vi "Odor_Control_b.vi"() -> ()   [LabVIEW 2014]
uses:
  <vilib>/Utility/file.llb/Read From Spreadsheet File (DBL).vi
  Image Aquisition - Labview/Image Recorder/experiment state global.vi
panel:
  in  "Sync Mode":bool
  out "Security Valve \nfor Mixtures":bool
  in  "threshold \nfor mixture":dbl
  in  "File with signal for odor 2":path=path "\\\\LABNAS40\\Luis/2016/Chemotaxis/Test/20160308/sine.txt"
  in  "File with signal for odor 1":path=path "\\\\LABNAS40\\Luis/2016/Chemotaxis/w1118_Acetal_1in250_50mfc/20160614/sine.txt"
  in  "ODOR 2":bool
  in  "ODOR 1":bool=TRUE
  in  "ODOR 2 FLOW %":dbl(slide) scale=0.0..100.0
  in  "ODOR 1 FLOW %":dbl(slide) scale=0.0..100.0
  in  "ODOR 2":bool
  in  "ODOR 1":bool=TRUE
  in  "TOLERANCE \nFOR CLOSING \nVALVE MANIFOLD":dbl=1.0
  in  "Serial Port":refnum<visa-resource-name>="COM3"
  in  "MODE SELECTOR":string(combo)="MANUAL"
  out "Path":path=path "B:/Luis/2016/0613/1047"
  in  "8":bool
  in  "7":bool
  in  "6":bool
  in  "5":bool
  in  "4":bool
  in  "3":bool
  in  "2":bool
  in  "1":bool
  in  "Start Recording":bool
  in  "extra label:":string="t101"
  in  "Save To:":path=path "B:/Luis"
  in  "CLEAR stored data":bool
  in  "Select signal to plot":T1(ring)=enum."odor 1 flow rate"
  out "XY Graph":T2(graph)
  in  "Air Flow Rate \n(L/min)":dbl
  in  "odor 2 between experiments":dbl
  in  "odor 2 signal parameters":T3={"temporal ramp type"=enum."Sine", "period(s)"=20.0, "high limit"=0.0, "low limit"=0.0, "duty cycle (sq wave)"=50.0} {"low limit" format="%#_6p"}
  in  "odor 1 between experiments":dbl
  in  "Sync Signal To \nImage Aquisition":bool
  in  "ENABLE MFCs":bool=TRUE
  in  "Restart Signal":bool
  in  "odor 1 signal parameters":T3={"temporal ramp type"=enum."Sine", "period(s)"=20.0, "high limit"=100.0, "low limit"=10.0, "duty cycle (sq wave)"=50.0} {"low limit" format="%#_6p"}
  in  "update period (ms)":u32=100
  in  "?":bool
  # "NOTE: Always start with Start Recording OFF, don't turn OFF while running"
  # "Manual Stop"
  # "VALVE CONTROL"
  # "MANUAL"
  # "FROM FILE"
  # "PREDEFINED WAVEFORM"
  # "PARAMETERS FOR BACKWASH PREVENTION"
  # "Only use when using odor \nmixture configuration, otherwise \nset to 0"
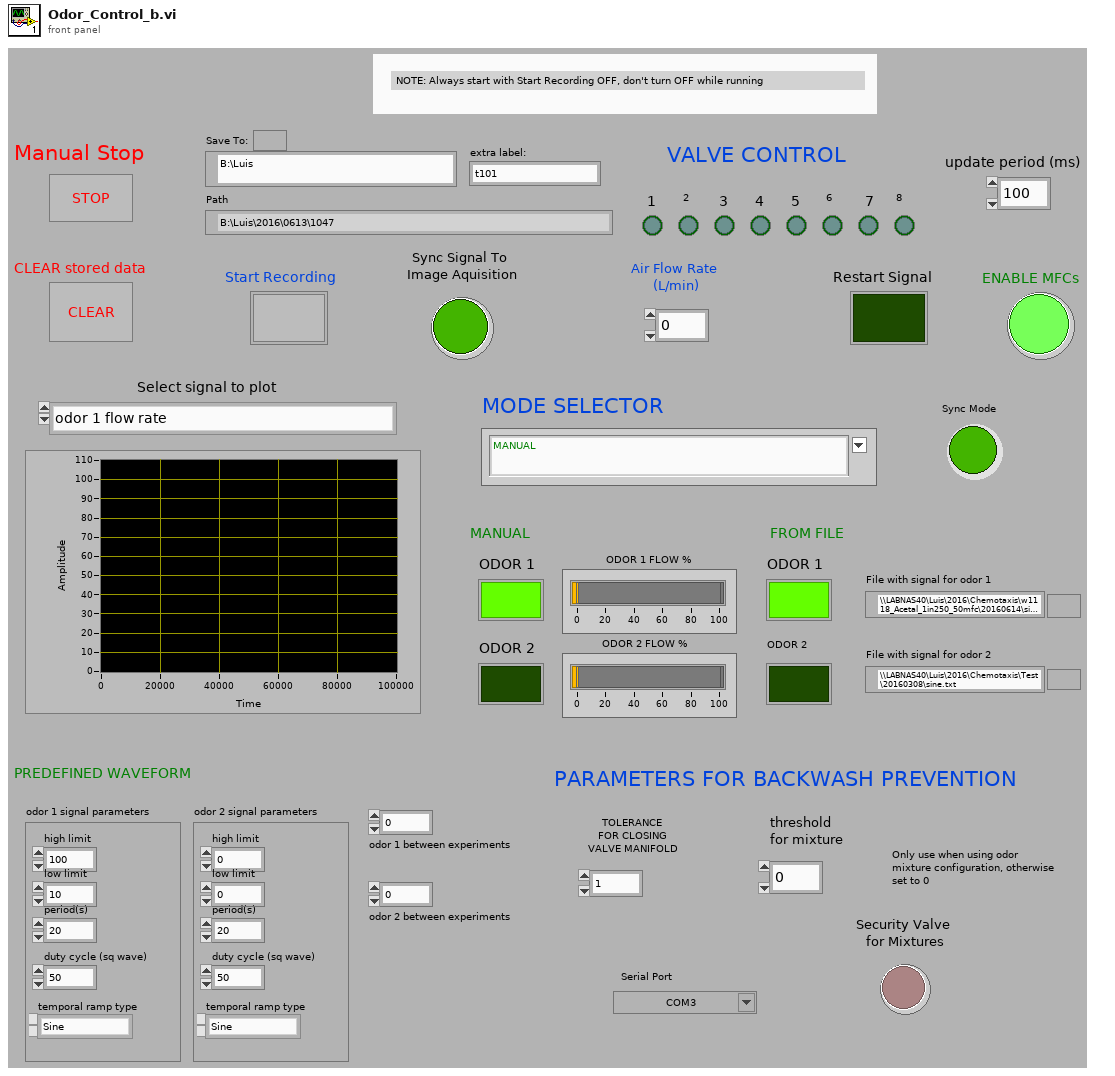
[diagram p1: front panel]
types:
  T1 = enum16{"air setpoint", "air flow rate", "odor 1 set point", "odor 1 flow rate", "odor 2 setpoint", "odor 2 flow rate", "pid reading", "led current", "led voltage", "led setpoint", "led temperature"}
  T2 = cluster{"Value Array":dbl[], "Value Array":dbl[]}
  T3 = cluster{"temporal ramp type":enum16{"Sine", "Triangle", "Sawtooth", "Square", "Exponential"}, "period(s)":dbl, "high limit":dbl, "low limit":dbl, "duty cycle (sq wave)":dbl}
  T4 = cluster{"analog output channels":cluster{"air ao":refnum<k21>, "odor 1 ao":refnum<k21>, "odor 2 ao":refnum<k21>}, "analog input channels":cluster{"air ai":refnum<k21>, "odor 1 ai":refnum<k21>, "odor 2 ai":refnum<k21>, "pid sensor 1 ai":refnum<k21>, "pid sensor 2 ai":refnum<k21>}, "digital control lines":cluster{"air close":refnum<k21>, "air purge":refnum<k21>, "odor 1 close":refnum<k21>, "odor 1 purge":refnum<k21>, "odor 2 close":refnum<k21>, "odor 2 purge":refnum<k21>}}
  T5 = enum16{"T - set Time per step", "N - set Number of valves", "F - turn gradient on Forward", "R - turn gradient on Reverse", "M - turn valves on 50% of time (mix)", "O - all valves Open (active)", "C - all valves Closed (inactive)", "V - set Valve state", "S - query valve State", "Q - Quiet (only error msgs)", "L - Loud (acknowledge all)", "H - useless Help message"}
  T6 = enum16{"Reset Table", "Get Values", "Add Value", "Get Table", "Get Spreadsheet", "set stack writer"}
  T7 = cluster{"experiment started":bool, "experiment ended":bool, "experiment start time":u32}
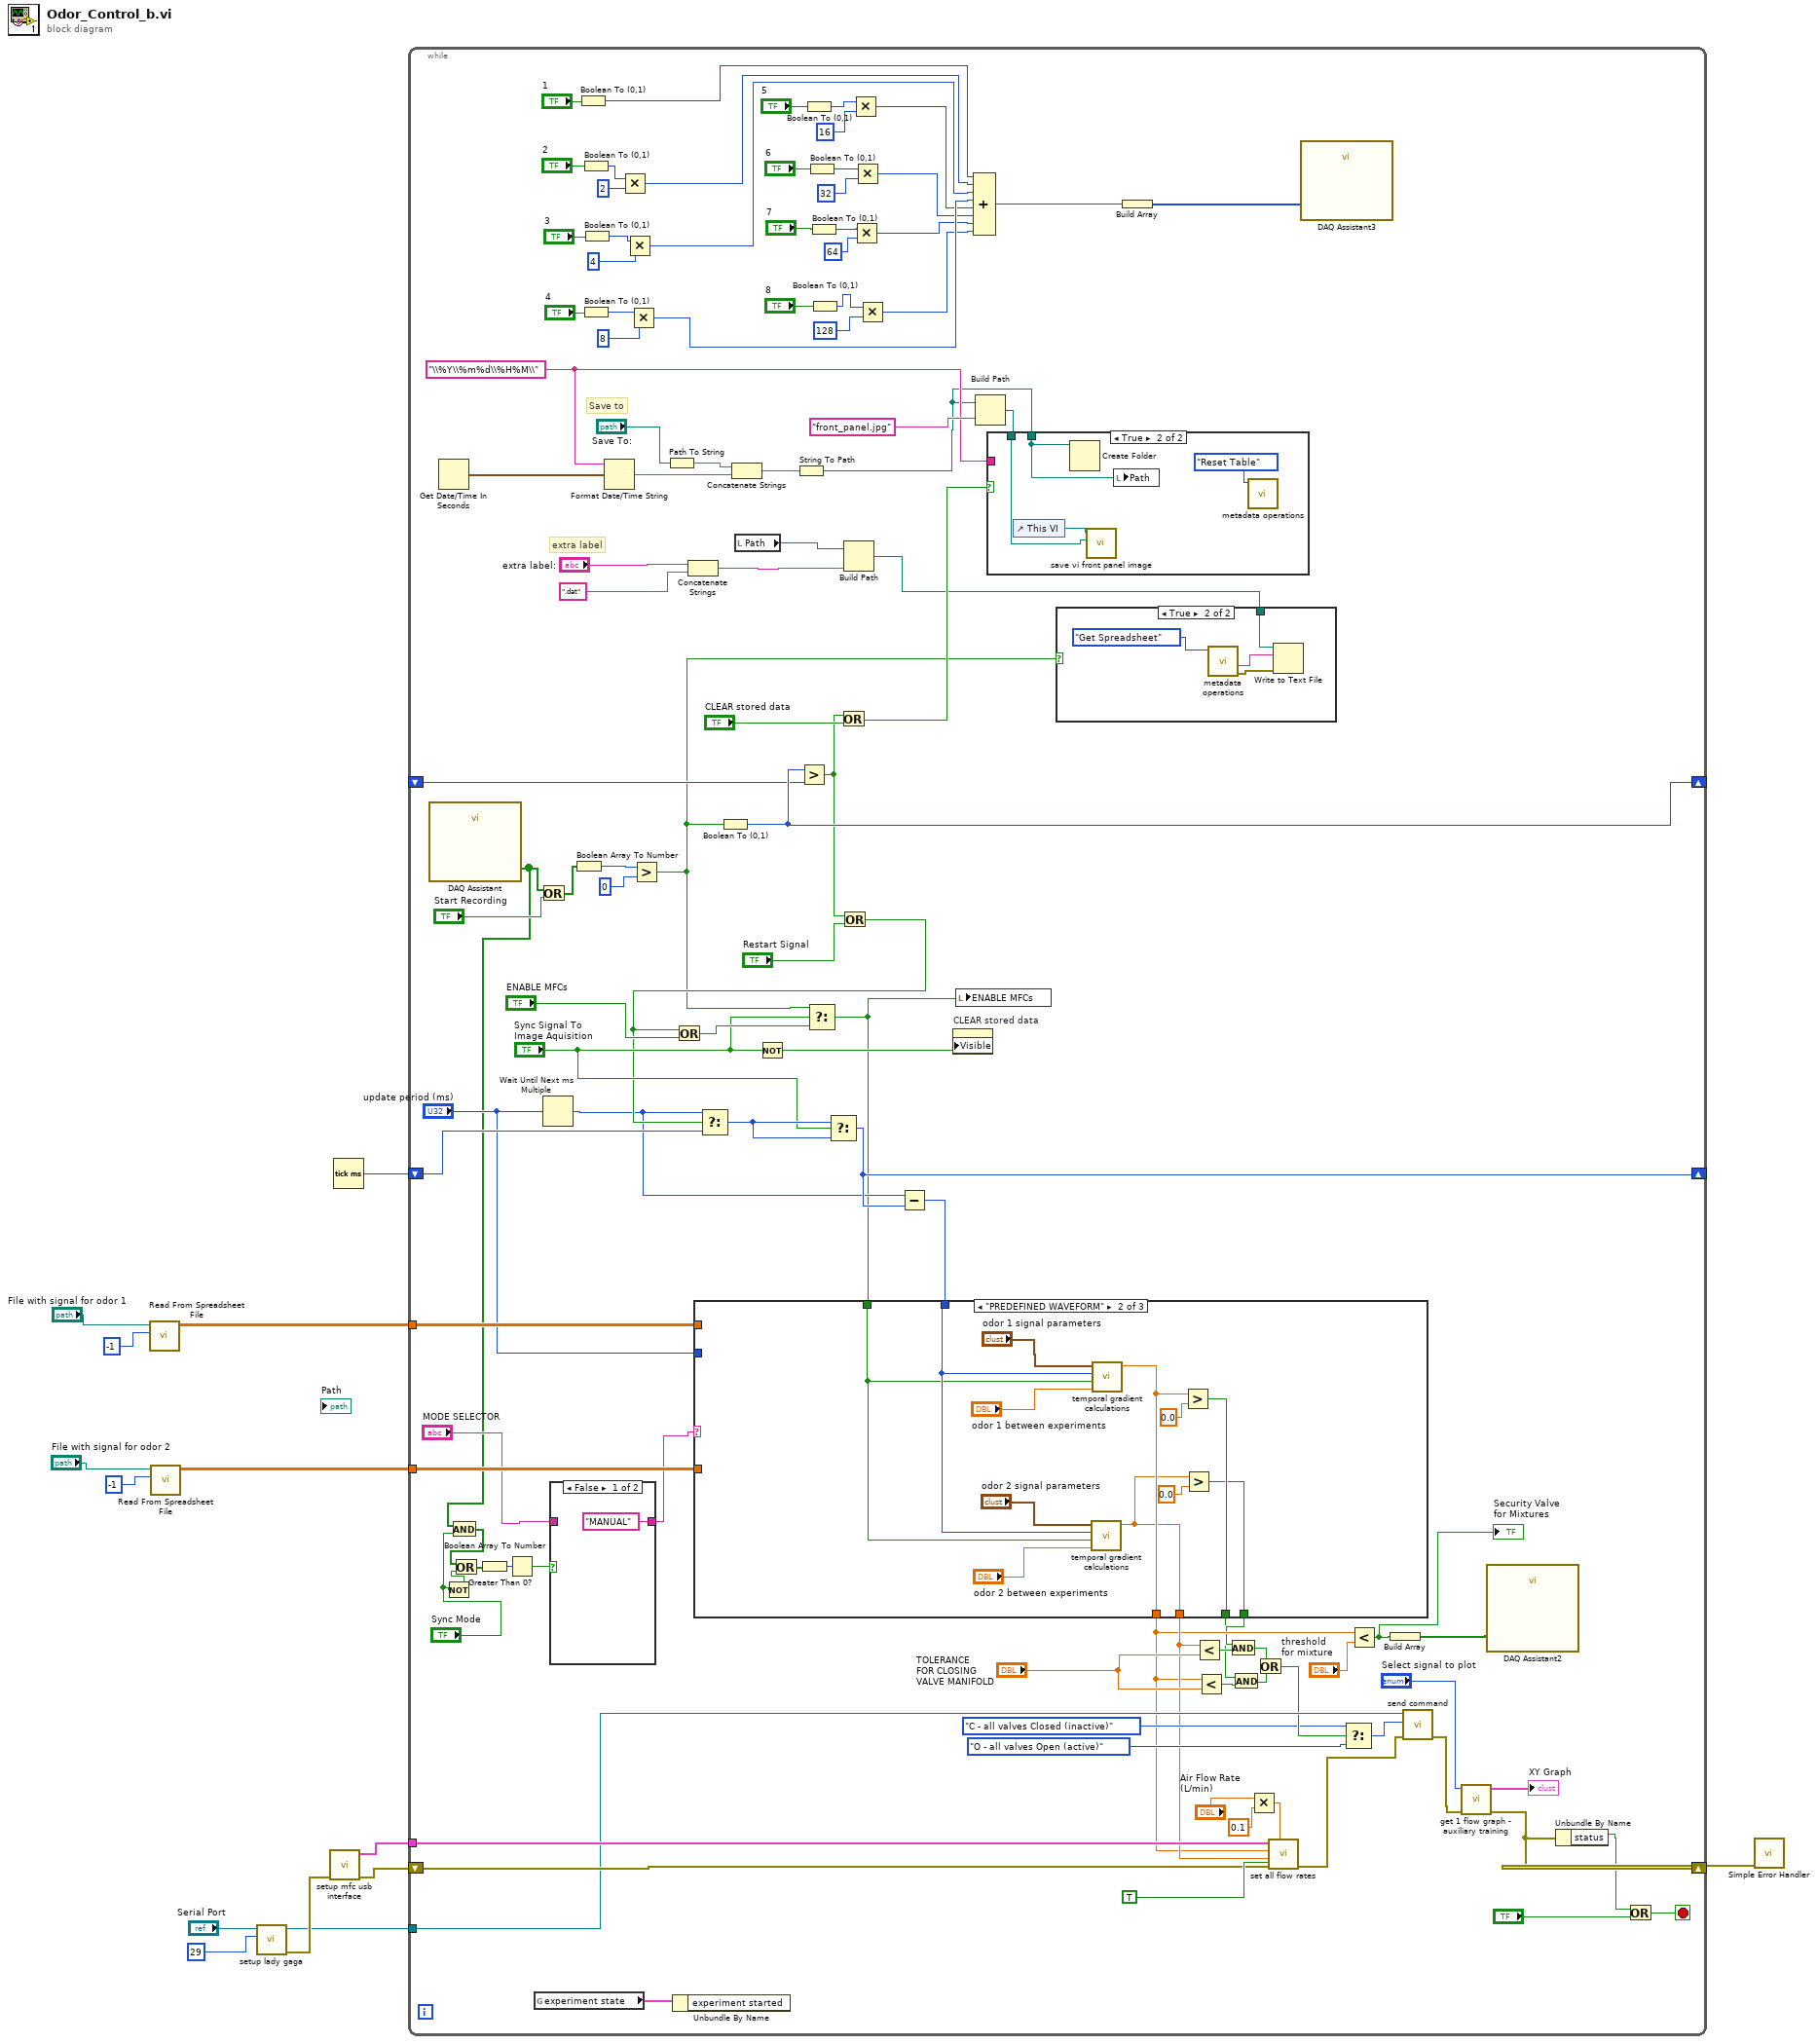
[diagram p0: block diagram]
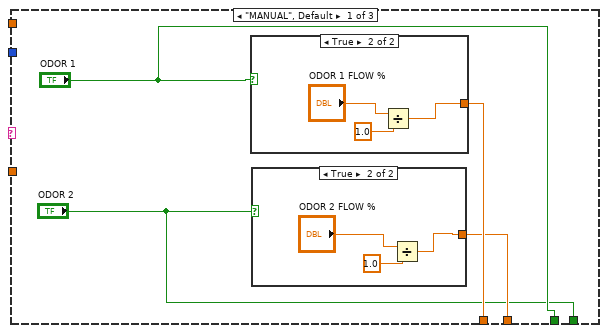
[diagram p3: hidden frame]
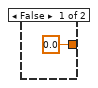
[diagram p4: hidden frame]
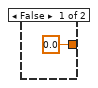
[diagram p5: hidden frame]
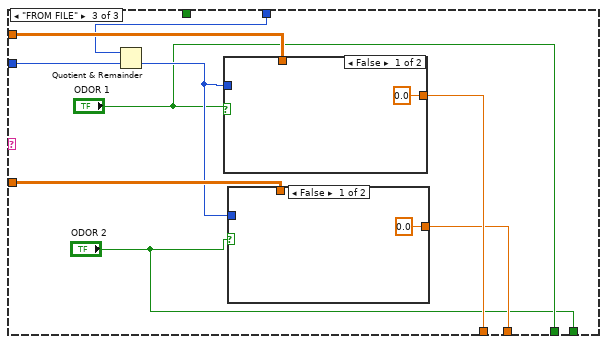
[diagram p6: hidden frame]
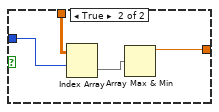
[diagram p7: hidden frame]
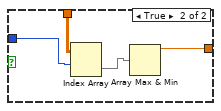
[diagram p8: hidden frame]
diagram:
  n1 = call-poly <vilib>:"Read From Spreadsheet File.vi"("number of rows (all:-1)"=-1, "file path (dialog if empty)"="File with signal for odor 1") -> ("all rows"=w2:dbl[][])  [unwired: 2 in, 7 out]
  n2 = call-poly <vilib>:"Read From Spreadsheet File.vi"("number of rows (all:-1)"=-1, "file path (dialog if empty)"="File with signal for odor 2") -> ("all rows"=w1:dbl[][])  [unwired: 2 in, 7 out]
  n3 = call "setup lady gaga.vi"("num valves"=u8 29, "LADY GAGA Serial Port Name"="Serial Port") -> ("error out"=w8:errorcluster, "LADY GAGA Serial Port"=w7:refnum<visa-resource-name>)  [unwired: 7 in, 1 out]
  n4 = call "setup mfc usb interface.vi"("error in"=w8) -> ("error out"=w13:errorcluster, "daqmx tasks"=w12:T4)  [unwired: 9 in]
  n5 = Tick Count (ms)() -> (millisecond timer value=w14:u32)
  n6 = while {
    shift-right: [w52] -> w11
    shift-left: w13 -> [w118]
    shift-right: [w123] -> _
    shift-left: w14 -> [w111]
    tunnel: w12 -> [w117]
    shift-right: [w108] -> _
    shift-left: _ -> [w107]
    tunnel: w7 -> [w48]
    tunnel: w2 -> [w40]
    tunnel: w1 -> [w39]
    stop <- w126 stop-if-true
    w56 = "\\%Y\\%m%d\\%H%M\\" ("time format string (%c)")
    # "extra label"
    # "Save to"
    n7 = call "DAQ Assistant"() -> ("data"=w18:bool[])  [unwired: 17 in, 2 out]
    n8 = Get Date/Time In Seconds() -> (seconds since 1Jan1904=w65:timestamp)
    n9 = Not(x="Sync Mode") -> (.not. x?=w16:bool)
    n10 = And(x=w18, y="Sync Mode") -> (x .and. y?=w17:bool[])
    n11 = Or(x=w17, y=w16) -> (x .or. y?=w19:bool[])
    n12 = Boolean Array To Number(Boolean array=w19) -> (number=w20:u32)
    n13 = Greater Than 0?(x=w20) -> (x > 0?=w21:bool)
    n14 = global read "experiment state global.vi" "experiment state"() -> (w120:T7)
    n15 = Or(x=w18, y="Start Recording") -> (x .or. y?=w102:bool[])
    n16 = Wait Until Next ms Multiple(millisecond multiple="update period (ms)") -> (millisecond timer value=w53:u32)
    n17 = case shown="False" w21 {
      tunnel: "MODE SELECTOR" -> [_ w128]
      tunnel: ["MANUAL" ("MODE SELECTOR") w128] -> w22
      frame False {
      }
      frame True {
      }
    }
    n18 = Boolean Array To Number(Boolean array=w102) -> (number=w113:u32)
    n19 = Boolean To (0,1)(Boolean="1") -> (0, 1=w79:i16)
    n20 = Boolean To (0,1)(Boolean="2") -> (0, 1=w93:i16)
    n21 = Boolean To (0,1)(Boolean="4") -> (0, 1=w91:i16)
    n22 = Boolean To (0,1)(Boolean="3") -> (0, 1=w92:i16)
    n23 = Format Date/Time String(time format string (%c)=w56, seconds (now)=w65) -> (date/time string=w62:string)  [unwired: 1 in]
    n24 = Multiply(x=w93, y=i16 2) -> (x*y=w78:i16)
    n25 = Multiply(x=w92, y=i16 4) -> (x*y=w77:i16)
    n26 = Multiply(x=w91, y=i16 8) -> (x*y=w76:i16)
    n27 = Greater?(x=w113, y=u32 0) -> (0:w54:bool)
    n28 = Path To String(path="Save To:") -> (string=w63:string)
    n29 = Unbundle By Name(w120) -> ()  [unwired: 1 out]
    n30 = Concatenate Strings("extra label:", ".dat" ("name or relative path")) -> (w60:string)
    n31 = Boolean To (0,1)(Boolean=w54) -> (0, 1=w108:i16)
    n32 = Concatenate Strings(w63, w62) -> (w61:string)
    n33 = local read "Path"() -> (w55:path)
    n34 = Not(x="Sync Signal To \nImage Aquisition") -> (.not. x?=w114:bool)
    n35 = String To Path(string=w61) -> (path=w51:path)
    n36 = Greater?(x=w108, y=w107) -> (0:w67:bool)
    n37 = Boolean To (0,1)(Boolean="5") -> (0, 1=w90:i16)
    n38 = Boolean To (0,1)(Boolean="6") -> (0, 1=w89:i16)
    n39 = Boolean To (0,1)(Boolean="7") -> (0, 1=w88:i16)
    n40 = Boolean To (0,1)(Boolean="8") -> (0, 1=w87:i16)
    n41 = Or(x=w67, y="CLEAR stored data") -> (x .or. y?=w105:bool)
    n42 = Or(x=w67, y="Restart Signal") -> (x .or. y?=w68:bool)
    n43 = Or(x=w68, y="ENABLE MFCs") -> (x .or. y?=w122:bool)
    n44 = Select(t=w53, s=w68, f=w111) -> (s? t:f=w110:u32)
    n45 = Select(t=w54, s="Sync Signal To \nImage Aquisition", f=w122) -> (s? t:f=w49:bool)
    n46 = Select(t=w110, s="Sync Signal To \nImage Aquisition", f=w110) -> (s? t:f=w123:u32)
    n47 = Build Path(base path=w55, name or relative path=w60) -> (appended path=w57:path)
    n48 = Multiply(x=w90, y=i16 16) -> (x*y=w75:i16)
    n49 = Multiply(x=w88, y=i16 64) -> (x*y=w73:i16)
    n50 = Multiply(x=w89, y=i16 32) -> (x*y=w74:i16)
    n51 = Multiply(x=w87, y=i16 128) -> (x*y=w72:i16)
    n52 = Subtract(x=w53, y=w123) -> (x-y=w50:u32)
    n53 = case shown="\"PREDEFINED WAVEFORM\"" w22 {
      tunnel: w50 -> [_ w148 w159]
      tunnel: w49 -> [_ w147 _]
      tunnel: [w131 w143 w155] -> w34
      tunnel: [w132 w146 w156] -> w30
      tunnel: w40 -> [_ _ w161]
      tunnel: w39 -> [_ _ w160]
      tunnel: "update period (ms)" -> [_ _ w158]
      tunnel: ["ODOR 1" w145 "ODOR 1"] -> w26
      tunnel: ["ODOR 2" w141 "ODOR 2"] -> w27
      frame "MANUAL", Default {
        n54 = case shown="True" "ODOR 1" {
          tunnel: [0.0 ("ODOR 1 FLOW %") w138] -> w132
          frame False {
          }
          frame True {
            n55 = Divide(x="ODOR 1 FLOW %", y=1.0) -> (x/y=w138:dbl)
          }
        }
        n56 = case shown="True" "ODOR 2" {
          tunnel: [0.0 ("ODOR 2 FLOW %") w134] -> w131
          frame False {
          }
          frame True {
            n57 = Divide(x="ODOR 2 FLOW %", y=1.0) -> (x/y=w134:dbl)
          }
        }
      }
      frame "PREDEFINED WAVEFORM" {
        n58 = call "temporal gradient calculations.vi"("grad disabled value"="odor 2 between experiments", "gradient enabled"=w147, "elapsed time (ms)"=w148, "gradient parameters"="odor 2 signal parameters") -> ("value"=w143:dbl)  [unwired: 7 in]
        n59 = call "temporal gradient calculations.vi"("grad disabled value"="odor 1 between experiments", "gradient enabled"=w147, "elapsed time (ms)"=w148, "gradient parameters"="odor 1 signal parameters") -> ("value"=w146:dbl)  [unwired: 7 in]
        n60 = Greater?(x=w146, y=0.0) -> (0:w145:bool)
        n61 = Greater?(x=w143, y=0.0) -> (0:w141:bool)
      }
      frame "FROM FILE" {
        n62 = Quotient & Remainder(x=w159, y=w158) -> (floor(x/y)=w157:u32)  [unwired: 1 out]
        n63 = case shown="False" "ODOR 1" {
          tunnel: w161 -> [_ w171]
          tunnel: w157 -> [_ w170]
          tunnel: [0.0 w168] -> w156
          frame False {
          }
          frame True {
            n64 = Index Array(array=w171, index (row)=w170) -> (element=w169:dbl[])  [unwired: 1 in]
            n65 = Array Max & Min(array=w169) -> (max value=w168:dbl)  [unwired: 3 out]
          }
        }
        n66 = case shown="False" "ODOR 2" {
          tunnel: w160 -> [_ w166]
          tunnel: w157 -> [_ w165]
          tunnel: [0.0 w163] -> w155
          frame False {
          }
          frame True {
            n67 = Index Array(array=w166, index (row)=w165) -> (element=w164:dbl[])  [unwired: 1 in]
            n68 = Array Max & Min(array=w164) -> (max value=w163:dbl)  [unwired: 3 out]
          }
        }
      }
    }
    n69 = property on="CLEAR stored data" class="Bool"("Visible"=w114) -> ()  [unwired: 2 in, 2 out]
    n70 = local write "ENABLE MFCs"(w49) -> ()
    n71 = Compound Arithmetic op=ADD(w79, w78, w77, w76, w75, w74, w73, w72) -> (w71:i16)
    n72 = Build Path(base path=w51, name or relative path="front_panel.jpg") -> (appended path=w58:path)
    n73 = case shown="True" w105 {
      tunnel: w51 -> [_ w176]
      tunnel: w58 -> [_ w178]
      tunnel: w56 -> [_ _]
      frame False {
      }
      frame True {
        n74 = control-ref of="This VI"() -> (w177:refnum<vi>)
        n75 = Create Folder(path (use dialog)=w176) -> ()  [unwired: 2 in, 3 out]
        n76 = call "save vi front panel image.vi"("path to JPEG file"=w178, "This VI"=w177) -> ()  [unwired: 9 in, 1 out]
        n77 = local write "Path"(w176) -> ()
        n78 = call "metadata operations.vi"("Operation"=T6."Reset Table") -> ()  [unwired: 7 in, 4 out]
      }
    }
    n79 = case shown="True" w54 {
      tunnel: w57 -> [_ w175]
      frame False {
      }
      frame True {
        n80 = call "metadata operations.vi"("Operation"=T6."Get Spreadsheet") -> ("error out"=w173:errorcluster, "spreadsheet table"=w172:string)  [unwired: 7 in, 2 out]
        n81 = Write to Text File(file (use dialog)=w175, text=w172, error in=w173) -> ()  [unwired: 1 in, 3 out]
      }
    }
    n82 = Build Array(w71) -> (w70:i16[])
    n83 = Less?(x=w34, y="TOLERANCE \nFOR CLOSING \nVALVE MANIFOLD") -> (x < y?=w29:bool)
    n84 = Less?(x=w30, y="TOLERANCE \nFOR CLOSING \nVALVE MANIFOLD") -> (x < y?=w28:bool)
    n85 = And(x=w27, y=w29) -> (x .and. y?=w25:bool)
    n86 = And(x=w26, y=w28) -> (x .and. y?=w24:bool)
    n87 = Multiply(x="Air Flow Rate \n(L/min)", y=0.1) -> (x*y=w35:dbl)
    n88 = Or(x=w25, y=w24) -> (x .or. y?=w46:bool)
    n89 = call "set all flow rates.vi"("log flow"=TRUE, "air flow rate"=w35, "error in"=w118, "odor 2 flow rate"=w34, "odor 1 flow rate"=w30, "daqmx tasks"=w117) -> ("error out"=w42:errorcluster)  [unwired: 5 in]
    n90 = call "DAQ Assistant3"("data"=w70) -> ()  [unwired: 17 in, 2 out]
    n91 = Select(t=T5."C - all valves Closed (inactive)" ("Command"), s=w46, f=T5."O - all valves Open (active)" ("Command")) -> (s? t:f=w43:T5)
    n92 = Less?(x=w30, y="threshold \nfor mixture") -> (x < y?=w31:bool)
    "Security Valve \nfor Mixtures" <- w31
    n93 = Build Array(w31) -> (w32:bool[])
    n94 = call "send command.vi"("error in"=w42, "Command"=w43, "LADY GAGA v2 Serial Port"=w48) -> ("error out"=w41:errorcluster)  [unwired: 5 in, 3 out]
    n95 = call "get 1 flow graph - auxiliary training.vi"("error in"=w41, "data to plot"="Select signal to plot") -> ("error out"=w52:errorcluster, "graph"=→"XY Graph":T2)  [unwired: 8 in]
    n96 = call "DAQ Assistant2"("data"=w32) -> ()  [unwired: 17 in, 2 out]
    n97 = Unbundle By Name(w52) -> ("status"=w124:bool)
    n98 = Or(x=w124, y="?") -> (x .or. y?=w126:bool)
  }
  n99 = call <vilib>:"Simple Error Handler.vi"("error in (no error)"=w11) -> ()  [unwired: 4 in, 5 out]
